vi "Execute schedule event.vi"(8 "ID":i32) -> ()   [LabVIEW 2018]
uses:
  Global variable.vi
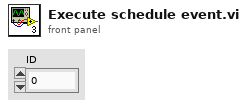
[diagram p1: front panel]
types:
  T1 = typedef "Schedule.ctl" = cluster{"Start time":timestamp, "Repeat":T2, "Action":T3}
  T2 = typedef "Repeat.ctl" = enum16{"None", "Every hour", "Every day", "Every week", "Every month"}
  T3 = typedef "Action.ctl" = u16
  T4 = typedef "LVDateTimeRec.ctl" = cluster{"fractional second":dbl, "second":i32, "minute":i32, "hour":i32, "day of month":i32, "month":i32, "year":i32, "day of week":i32, "day of year":i32, "DST":i32}
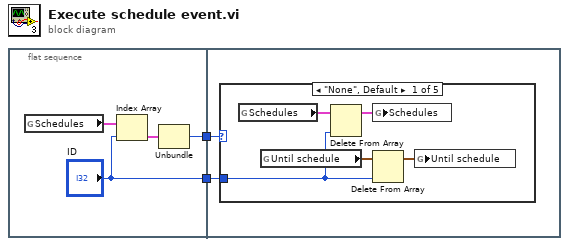
[diagram p0: block diagram]
diagram:
  n1 = flat-sequence {
    tunnel: ["ID"] -> w2
    tunnel: [w3] -> w1
    tunnel: w2 -> [w8]
    tunnel: w1 -> [w7]
    frame #0 {
      n2 = global read "Global variable.vi" "Schedules"() -> (w6:T1[])
      n3 = Index Array(array=w6, index="ID") -> (element=w5:T1)
      n4 = Unbundle(w5) -> ("Repeat"=w3:T2)  [unwired: 2 out]
    }
    frame #1 {
      n5 = case shown="\"None\", Default" w7 {
        tunnel: w8 -> [w11 _ _ _ _]
        frame "None", Default {
          n6 = global read "Global variable.vi" "Schedules"() -> (w12:T1[])
          n7 = global read "Global variable.vi" "Until schedule"() -> (w10:T4[])
          n8 = Delete From Array(array=w12, index=w11) -> (array with subset deleted=w13:T1[])  [unwired: 1 in, 1 out]
          n9 = global write "Global variable.vi" "Schedules"(w13) -> ()
          n10 = Delete From Array(array=w10, index=w11) -> (array with subset deleted=w9:T4[])  [unwired: 1 in, 1 out]
          n11 = global write "Global variable.vi" "Until schedule"(w9) -> ()
        }
        frame "Every hour" {
        }
        frame "Every day" {
        }
        frame "Every week" {
        }
        frame "Every month" {
        }
      }
    }
  }
